vi "4461 - Create AO waveforms.vi"(6 "sampling":T8={"Fs"=204789.0, "#s"=15753}, 8 "error in (no error)":errorcluster, 10 "reset signal":bool, 11 "AO":T1={"AO Amp (V)"=[0.1, 0.09, 0.08, 0.07, 0.06, 0.05, 0.04, 0.03], "AO DC (V)"=[0.0, 0.0, 0.0, 0.0, 0.0, 0.0, 0.0, 0.0], "AO f (Hz)"=[13.0, 13.0, 13.0, 13.0, 13.0, 13.0, 13.0, 13.0], "AO Phase (°)"=[0.0, 0.0, 0.0, 0.0, 0.0, 0.0, 0.0, 0.0], "Function"=[enum."Sine", enum."Sine", enum."Sine", enum."Sine", enum."Sine", enum."Sine", enum."Sine", enum."Sine"], "I+"=[], "Sweeping"=[]} {"AO f (Hz)" min=0.001 max=10000.0; "AO DC (V)" format="%.3p"; "AO Amp (V)" format="%.3p"}) -> (0 "error out":errorcluster, 1 "phase out":dbl[](array[numeric]), 2 "AO Array":waveform(dbl)[](array[waveform]), 3 "AO 2":T1={"AO Amp (V)"=[0.1, 0.09, 0.08, 0.07, 0.06, 0.05, 0.04, 0.03], "AO DC (V)"=[0.0, 0.0, 0.0, 0.0, 0.0, 0.0, 0.0, 0.0], "AO f (Hz)"=[13.0, 13.0, 13.0, 13.0, 13.0, 13.0, 13.0, 13.0], "AO Phase (°)"=[0.0, 0.0, 0.0, 0.0, 0.0, 0.0, 0.0, 0.0], "Function"=[enum."Sine", enum."Sine", enum."Sine", enum."Sine", enum."Sine", enum."Sine", enum."Sine", enum."Sine"], "I+"=[], "Sweeping"=[]} {"AO f (Hz)" min=0.001 max=10000.0; "AO DC (V)" format="%.3p"; "AO Amp (V)" format="%.3p"})   [LabVIEW 2016, in "Instrument.Lockin.lvclass"]
uses:
  Instrument.Lockin.lvclass
  Typedefs/Sampling.ctl
  Typedefs/AO-cluster.ctl
  Typedefs/AO_Amp-array.ctl
  Typedefs/AO_DC-array.ctl
  Typedefs/AO_f-array.ctl
  Typedefs/AO_phi-array.ctl
  Typedefs/Function-array.ctl
  Typedefs/Function-enum.ctl
  <vilib>/measure/NI_MABase.lvlib
panel:
  out "Waveform Chart":dbl[][](graph)
  out "Waveform Graph 2":waveform(dbl)[](graph)
  out "Numeric":i32
  # "1"
  # "2"
  # "3"
  # "4"
  # "5"
  # "6"
  # "7"
  # "8"
  # "1"
  # "2"
  # "3"
  # "4"
  # "5"
  # "6"
  # "7"
  # "8"
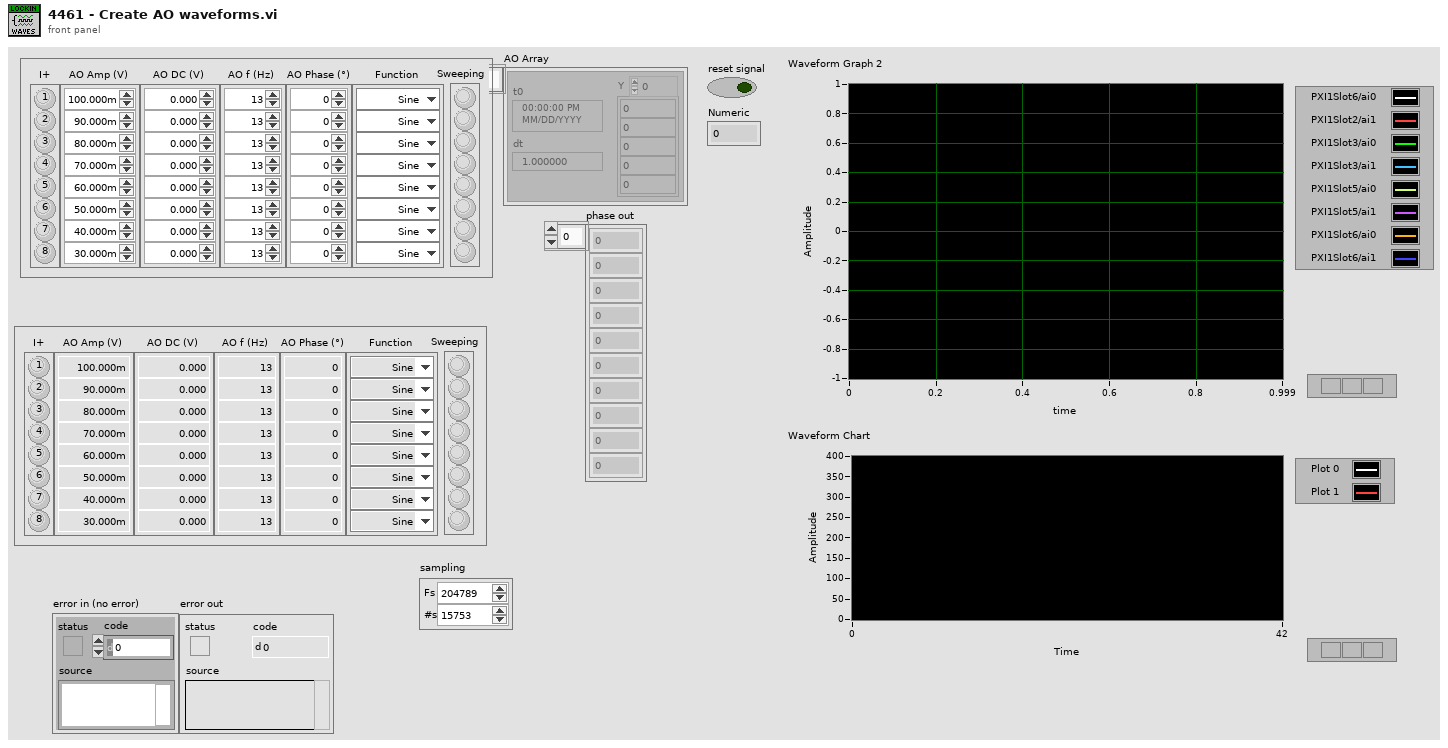
[diagram p1: front panel]
types:
  T1 = typedef "Instrument.Lockin.lvclass/AO-cluster.ctl" = cluster{"AO Amp (V)":T2, "AO DC (V)":T3, "AO f (Hz)":T4, "AO Phase (°)":T5, "Function":T6, "I+":bool[], "Sweeping":bool[]}
  T2 = typedef "Instrument.Lockin.lvclass/AO_Amp-array.ctl" = dbl[]
  T3 = typedef "Instrument.Lockin.lvclass/AO_DC-array.ctl" = dbl[]
  T4 = typedef "Instrument.Lockin.lvclass/AO_f-array.ctl" = dbl[]
  T5 = typedef "Instrument.Lockin.lvclass/AO_phi-array.ctl" = dbl[]
  T6 = typedef "Instrument.Lockin.lvclass/Function-array.ctl" = T7[]
  T7 = typedef "Instrument.Lockin.lvclass/Function-enum.ctl" = enum16{"Sine", "Triangle", "Square", "Sawtooth"}
  T8 = typedef "Instrument.Lockin.lvclass/Sampling.ctl" = cluster{"Fs":dbl, "#s":i32}
  T9 = enum16{"Sine Wave", "Triangle Wave", "Square Wave", "Sawtooth Wave"}
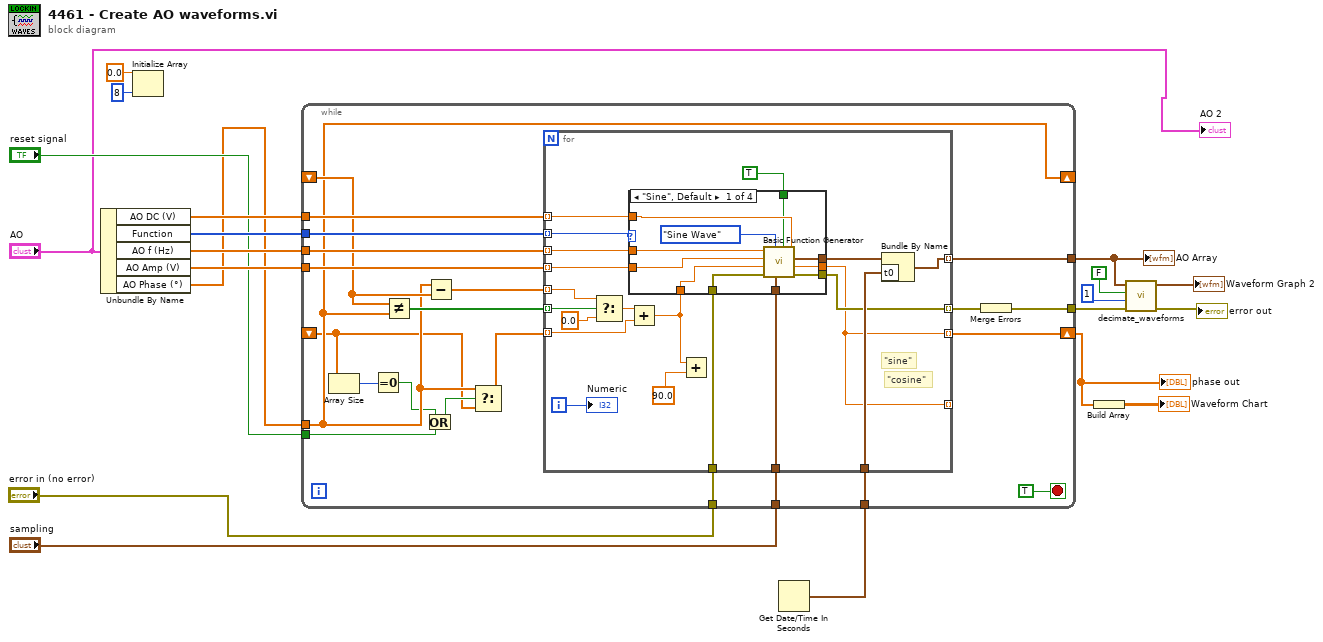
[diagram p0: block diagram]
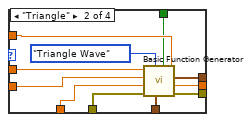
[diagram p2: hidden frame]
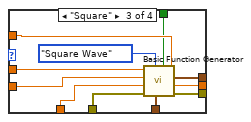
[diagram p3: hidden frame]
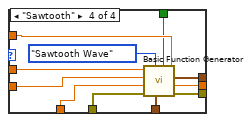
[diagram p4: hidden frame]
diagram:
  n1 = Unbundle By Name("AO") -> ("AO DC (V)"=w19:T3, "Function"=w20:T6, "AO f (Hz)"=w16:T4, "AO Amp (V)"=w17:T2, "AO Phase (°)"=w3:T5)
  n2 = Initialize Array(0.0 ("element"), 8 ("dimension size")) -> ()  [unwired: 1 out]
  n3 = Get Date/Time In Seconds() -> (seconds since 1Jan1904=w1:timestamp)
  n4 = while {
    tunnel: w20 -> [w42]
    tunnel: w19 -> [w41]
    tunnel: "sampling" -> [w40]
    tunnel: [w39] -> w12
    tunnel: w17 -> [w38]
    tunnel: w3 -> [w29]
    tunnel: w16 -> [w37]
    shift-right: [w29] -> _
    shift-left: _ -> [w34]
    shift-right: [w32] -> w6
    shift-left: _ -> [w21]
    tunnel: w1 -> [w31]
    tunnel: "reset signal" -> [w26]
    tunnel: "error in (no error)" -> [w24]
    tunnel: [w22] -> w9
    stop <- TRUE stop-if-true
    n5 = Array Size(array=w21) -> (size(s)=w30:i32)
    n6 = Equal To 0?(x=w30) -> (x = 0?=w27:bool)
    n7 = Not Equal?(x=w34, y=w29) -> (x != y?=w35:bool[])
    n8 = Or(x=w27, y=w26) -> (x .or. y?=w28:bool)
    n9 = Subtract(x=w29, y=w34) -> (x-y=w33:T5)
    n10 = Select(t=w29, s=w28, f=w21) -> (s? t:f=w25:T5)
    n11 = for {
      tunnel: w42 -> [w43] mode=indexing
      tunnel: w37 -> [w62] mode=indexing
      tunnel: w38 -> [w46] mode=indexing
      tunnel: w41 -> [w61] mode=indexing
      tunnel: [w51] -> w39 mode=indexing
      tunnel: w40 -> [w44]
      tunnel: w35 -> [w55] mode=indexing
      tunnel: w33 -> [w57] mode=indexing
      tunnel: [w48] -> w32 mode=indexing
      tunnel: w25 -> [w47] mode=indexing
      tunnel: w31 -> [w54]
      tunnel: [w48] -> _ mode=indexing
      tunnel: w24 -> [w50]
      tunnel: [w49] -> w23 mode=indexing
      i -> [w53]
      # "\"cosine\""
      # "\"sine\""
      n12 = Select(t=w57, s=w55, f=0.0) -> (s? t:f=w58:dbl)
      n13 = Add(x=w58, y=w47) -> (x+y=w45:dbl)
      n14 = case shown="\"Sine\", Default" w43 {
        tunnel: w62 -> [w73 w84 w95 w106]
        tunnel: w61 -> [w72 w83 w94 w105]
        tunnel: [w71 w82 w93 w104] -> w60
        tunnel: TRUE ("reset signal") -> [w70 w81 w92 w103]
        tunnel: w50 -> [w69 w80 w91 w102]
        tunnel: [w68 w79 w90 w101] -> w49
        tunnel: [w67 w78 w89 w100] -> w48
        tunnel: w46 -> [w66 w77 w88 w99]
        tunnel: w45 -> [w65 w76 w87 w98]
        tunnel: w44 -> [w64 w75 w86 w97]
        frame "Sine", Default {
          n15 = call <vilib>:"Basic Function Generator.vi"("offset"=w72, "reset signal"=w70, "sampling info"=w64, "signal type"=T9."Sine Wave", "error in (no error)"=w69, "phase"=w65, "amplitude"=w66, "frequency"=w73) -> ("error out"=w68:errorcluster, "phase out"=w67:dbl, "signal out"=w71:waveform(dbl))  [unwired: 1 in]
        }
        frame "Triangle" {
          n16 = call <vilib>:"Basic Function Generator.vi"("offset"=w83, "reset signal"=w81, "sampling info"=w75, "signal type"=T9."Triangle Wave", "error in (no error)"=w80, "phase"=w76, "amplitude"=w77, "frequency"=w84) -> ("error out"=w79:errorcluster, "phase out"=w78:dbl, "signal out"=w82:waveform(dbl))  [unwired: 1 in]
        }
        frame "Square" {
          n17 = call <vilib>:"Basic Function Generator.vi"("offset"=w94, "reset signal"=w92, "sampling info"=w86, "signal type"=T9."Square Wave", "error in (no error)"=w91, "phase"=w87, "amplitude"=w88, "frequency"=w95) -> ("error out"=w90:errorcluster, "phase out"=w89:dbl, "signal out"=w93:waveform(dbl))  [unwired: 1 in]
        }
        frame "Sawtooth" {
          n18 = call <vilib>:"Basic Function Generator.vi"("offset"=w105, "reset signal"=w103, "sampling info"=w97, "signal type"=T9."Sawtooth Wave", "error in (no error)"=w102, "phase"=w98, "amplitude"=w99, "frequency"=w106) -> ("error out"=w101:errorcluster, "phase out"=w100:dbl, "signal out"=w104:waveform(dbl))  [unwired: 1 in]
        }
      }
      n19 = Add(x=w45, y=90.0) -> ()  [unwired: 1 out]
      n20 = Bundle By Name(cluster=w60, "t0"=w54) -> (w51:waveform(dbl))
      "Numeric" <- w53
    }
    n21 = Merge Errors(w23) -> (w22:errorcluster)
  }
  "AO Array" <- w12
  "phase out" <- w6
  n22 = Build Array(w6) -> (→"Waveform Chart":dbl[][])
  n23 = call "decimate_waveforms.vi"("Input Signal"=w12, "averaging"=FALSE, "decimating factor"=1, "error in (no error)"=w9) -> ("Decimated Waveforms"=→"Waveform Graph 2":waveform(dbl)[], "error out"=→"error out":errorcluster)  [unwired: 5 in]
  "AO 2" <- "AO"
